vi "niusrprios Open and Configure Device.vi"(0 "USRP RIO Device":T16, 5 "reference frequency source":string(combo)="Internal", 7 "which bitfile":string(combo)="Time", 9 "Wait for GPS Lock?":bool, 11 "error in":errorcluster, 12 "rx config":T4={"rf enable 0"=FALSE, "rf config 0"={"antenna"="RX2", "frequency"=2000000000.0, "lo frequency"=-1.0, "level"=0.0}, "rf enable 1"=FALSE, "rf config 1"={"antenna"="RX2", "frequency"=2000000000.0, "lo frequency"=-1.0, "level"=0.0}, "transfer mode"=enum."Finite", "sample rate"=10000000.0, "number of samples"=8192, "start trigger"=enum."Immediate"} {"sample rate" format="%#.3pS/s"; "rf config 1"."level" format="%#_gdBm"; "rf config 1"."lo frequency" format="%#.3pHz"; "rf config 1"."frequency" format="%#.3pHz"; "rf config 0"."level" format="%#_gdBm"; "rf config 0"."lo frequency" format="%#.3pHz"; "rf config 0"."frequency" format="%#.3pHz"}, 13 "tx config":T5={"rf enable 0"=FALSE, "rf config 0"={"antenna"="TX1", "frequency"=2000000000.0, "lo frequency"=-1.0, "level"=0.0}, "rf enable 1"=FALSE, "rf config 1"={"antenna"="TX1", "frequency"=2000000000.0, "lo frequency"=-1.0, "level"=0.0}, "transfer mode"=enum."Finite", "sample rate"=10000000.0, "number of samples"=8192, "start trigger"=enum."Immediate", "tone frequency"=100000.0} {"tone frequency" format="%#.3pHz"; "sample rate" format="%#.3pS/s"; "rf config 0"."level" format="%#_gdBm"; "rf config 0"."lo frequency" format="%#.3pHz"; "rf config 0"."frequency" format="%#.3pHz"; "rf config 1"."level" format="%#_gdBm"; "rf config 1"."lo frequency" format="%#.3pHz"; "rf config 1"."frequency" format="%#.3pHz"}) -> (2 "rx channels":T3={"rx config"={"rf enable 0"=FALSE, "rf config 0"={"antenna"="RX2", "frequency"=2000000000.0, "lo frequency"=-1.0, "level"=0.0}, "rf enable 1"=FALSE, "rf config 1"={"antenna"="RX2", "frequency"=2000000000.0, "lo frequency"=-1.0, "level"=0.0}, "transfer mode"=enum."Finite", "sample rate"=10000000.0, "number of samples"=8192, "start trigger"=enum."Immediate"}, "reference frequency source"="Internal", "rx.enabled channels"=[], "vertical range"=[], "rx.coerced configurations"={"coerced frequencies"=[], "coerced lo frequencies"=[], "coerced levels"=[], "coerced sample rates"=[]}} {"rx.coerced configurations"."coerced sample rates" format="%#.3pS/s"; "rx.coerced configurations"."coerced levels" format="%#.3gdBm"; "rx.coerced configurations"."coerced lo frequencies" format="%#.3pHz"; "rx.coerced configurations"."coerced frequencies" format="%#.3pHz"; "rx config"."sample rate" format="%#.3pS/s"; "rx config"."rf config 1"."level" format="%#_gdBm"; "rx config"."rf config 1"."lo frequency" format="%#.3pHz"; "rx config"."rf config 1"."frequency" format="%#.3pHz"; "rx config"."rf config 0"."level" format="%#_gdBm"; "rx config"."rf config 0"."lo frequency" format="%#.3pHz"; "rx config"."rf config 0"."frequency" format="%#.3pHz"; "vertical range" format="%#.3pVpp"}, 3 "tx channels":T2={"tx config"={"rf enable 0"=FALSE, "rf config 0"={"antenna"="TX1", "frequency"=2000000000.0, "lo frequency"=-1.0, "level"=0.0}, "rf enable 1"=FALSE, "rf config 1"={"antenna"="TX1", "frequency"=2000000000.0, "lo frequency"=-1.0, "level"=0.0}, "transfer mode"=enum."Finite", "sample rate"=10000000.0, "number of samples"=8192, "start trigger"=enum."Immediate", "tone frequency"=100000.0}, "reference frequency source"="Internal", "tx.enabled channels"=[], "I"=[], "Q"=[], "tx.coerced configurations"={"coerced frequencies"=[], "coerced lo frequencies"=[], "coerced levels"=[], "coerced sample rates"=[]}} {"tx.coerced configurations"."coerced sample rates" format="%#.3pS/s"; "tx.coerced configurations"."coerced levels" format="%#.3gdBm"; "tx.coerced configurations"."coerced lo frequencies" format="%#.3pHz"; "tx.coerced configurations"."coerced frequencies" format="%#.3pHz"; "tx config"."tone frequency" format="%#.3pHz"; "tx config"."sample rate" format="%#.3pS/s"; "tx config"."rf config 0"."level" format="%#_gdBm"; "tx config"."rf config 0"."lo frequency" format="%#.3pHz"; "tx config"."rf config 0"."frequency" format="%#.3pHz"; "tx config"."rf config 1"."level" format="%#_gdBm"; "tx config"."rf config 1"."lo frequency" format="%#.3pHz"; "tx config"."rf config 1"."frequency" format="%#.3pHz"}, 4 "niUsrpRio Session (out)":T7 {"Daughterboard Clock Rate" format="%#.3pHz"; "FPGA Data Clock Rate" format="%#.3pHz"; "Data Clock Rate" format="%#.3pHz"; "Characterization Data"."Frequencies [Hz]" format="%#_6p"; "EEPROM Characterization Header"."Pointer to Device Data Header" format="%x"; "EEPROM Characterization Header"."Checksum" format="%x"; "Device Data Header"."Pointer to Characterization Data" format="%x"; "Device Data Header"."Checksum" format="%x"; "EEPROM Header"."Pointer to User Header" format="%x"; "EEPROM Header"."Pointer to Factory Header" format="%x"; "EEPROM Header"."Product Code" format="%x"; "EEPROM Header"."Checksum" format="%x"}, 6 "rx.coerced configurations":T6 {"coerced sample rates" format="%#.3pS/s"; "coerced levels" format="%#.3gdBm"; "coerced lo frequencies" format="%#.3pHz"; "coerced frequencies" format="%#.3pHz"}, 8 "tx.coerced configurations":T6 {"coerced sample rates" format="%#.3pS/s"; "coerced levels" format="%#.3gdBm"; "coerced lo frequencies" format="%#.3pHz"; "coerced frequencies" format="%#.3pHz"}, 10 "tx.output waveform":waveform(dbl)[](graph), 15 "error out":errorcluster)   [LabVIEW 2015]
doc: "Opens a session to the USRP RIO design library, initializes the device and configures the RF components.\n\n<B>Input Parameters</B>\n\n<B>USRP RIO device</B> is the specific device to open a session to.\n\n<B>reference frequency source</B> is the reference source to use for the clocks of the device. The reference frequency must be 10 MHz.\n\n<B>error in</B> describes error conditions that occur before this node runs. This input provides standard 'error in' functionality.\n\n<B>rx config</B> is the set of configuration values for the Rx signal chain.\n\n<B>tx config</B> is the set of configuration values for the Tx signal chain.\n\n<B>Output Parameters</B>\n\n<B>niUsrpRio Session (out)</B> is the niUsrpRio session used in all subsequent USRP RIO design library host VIs.\n\n<B>rx.coerced configurations</B> are the actual configuration values for the Rx signal chain.\n\n<B>tx.coerced configurations</B> are the actual configuration values for the Tx signal chain.\n\n<B>tx.output waveform</B> is the baseband signal to use when transmitting.\n\n<B>error out</B> contains error information. This output provides standard 'error out' functionality."
uses:
  <vilib>/userdefined/Silver/nirio_resource_slv.ctl
  <instrlib>/niUsrpRio/Config/v1/Host/Public/niUsrpRio Session.ctl
  <instrlib>/_niInstr/Register Bus/v0/Host/Public/Register Bus Session.ctl
  <instrlib>/_niInstr/Register Bus/v0/Host/Private/Session Data.ctl
  <instrlib>/niUsrpRio/Config/v1/Host/Private/DB Queue Reference.ctl
  <instrlib>/niUsrpRio/Config/v1/Host/Private/Daughterboard Data.ctl
  <instrlib>/niUsrpRio/Config/v1/Host/Private/ATR state data.ctl
  <instrlib>/niUsrpRio/Config/v1/Host/Private/Antenna Configuration.ctl
  <instrlib>/niUsrpRio/Config/v1/Host/Private/CPLD Power Mode.ctl
  <instrlib>/niUsrpRio/Config/v1/Host/Public/EEPROM Header.ctl
  <instrlib>/niUsrpRio/Config/v1/Host/Public/EEPROM Device Data Header.ctl
  <instrlib>/niUsrpRio/Config/v1/Host/Public/EEPROM Characterization Header.ctl
  <instrlib>/niUsrpRio/Config/v1/Host/Public/Characterization Data.ctl
  <instrlib>/niUsrpRio/Config/v1/Host/Public/IQ Imbalance.ctl
  niusrprios Start Trigger.ctl
  <instrlib>/_niInstr/Register Bus/v0/Host/niInstr Register Bus v0 Host.lvlib
  <instrlib>/niUsrpRio/Config/v1/Host/niUsrpRio Config v1 Host.lvlib
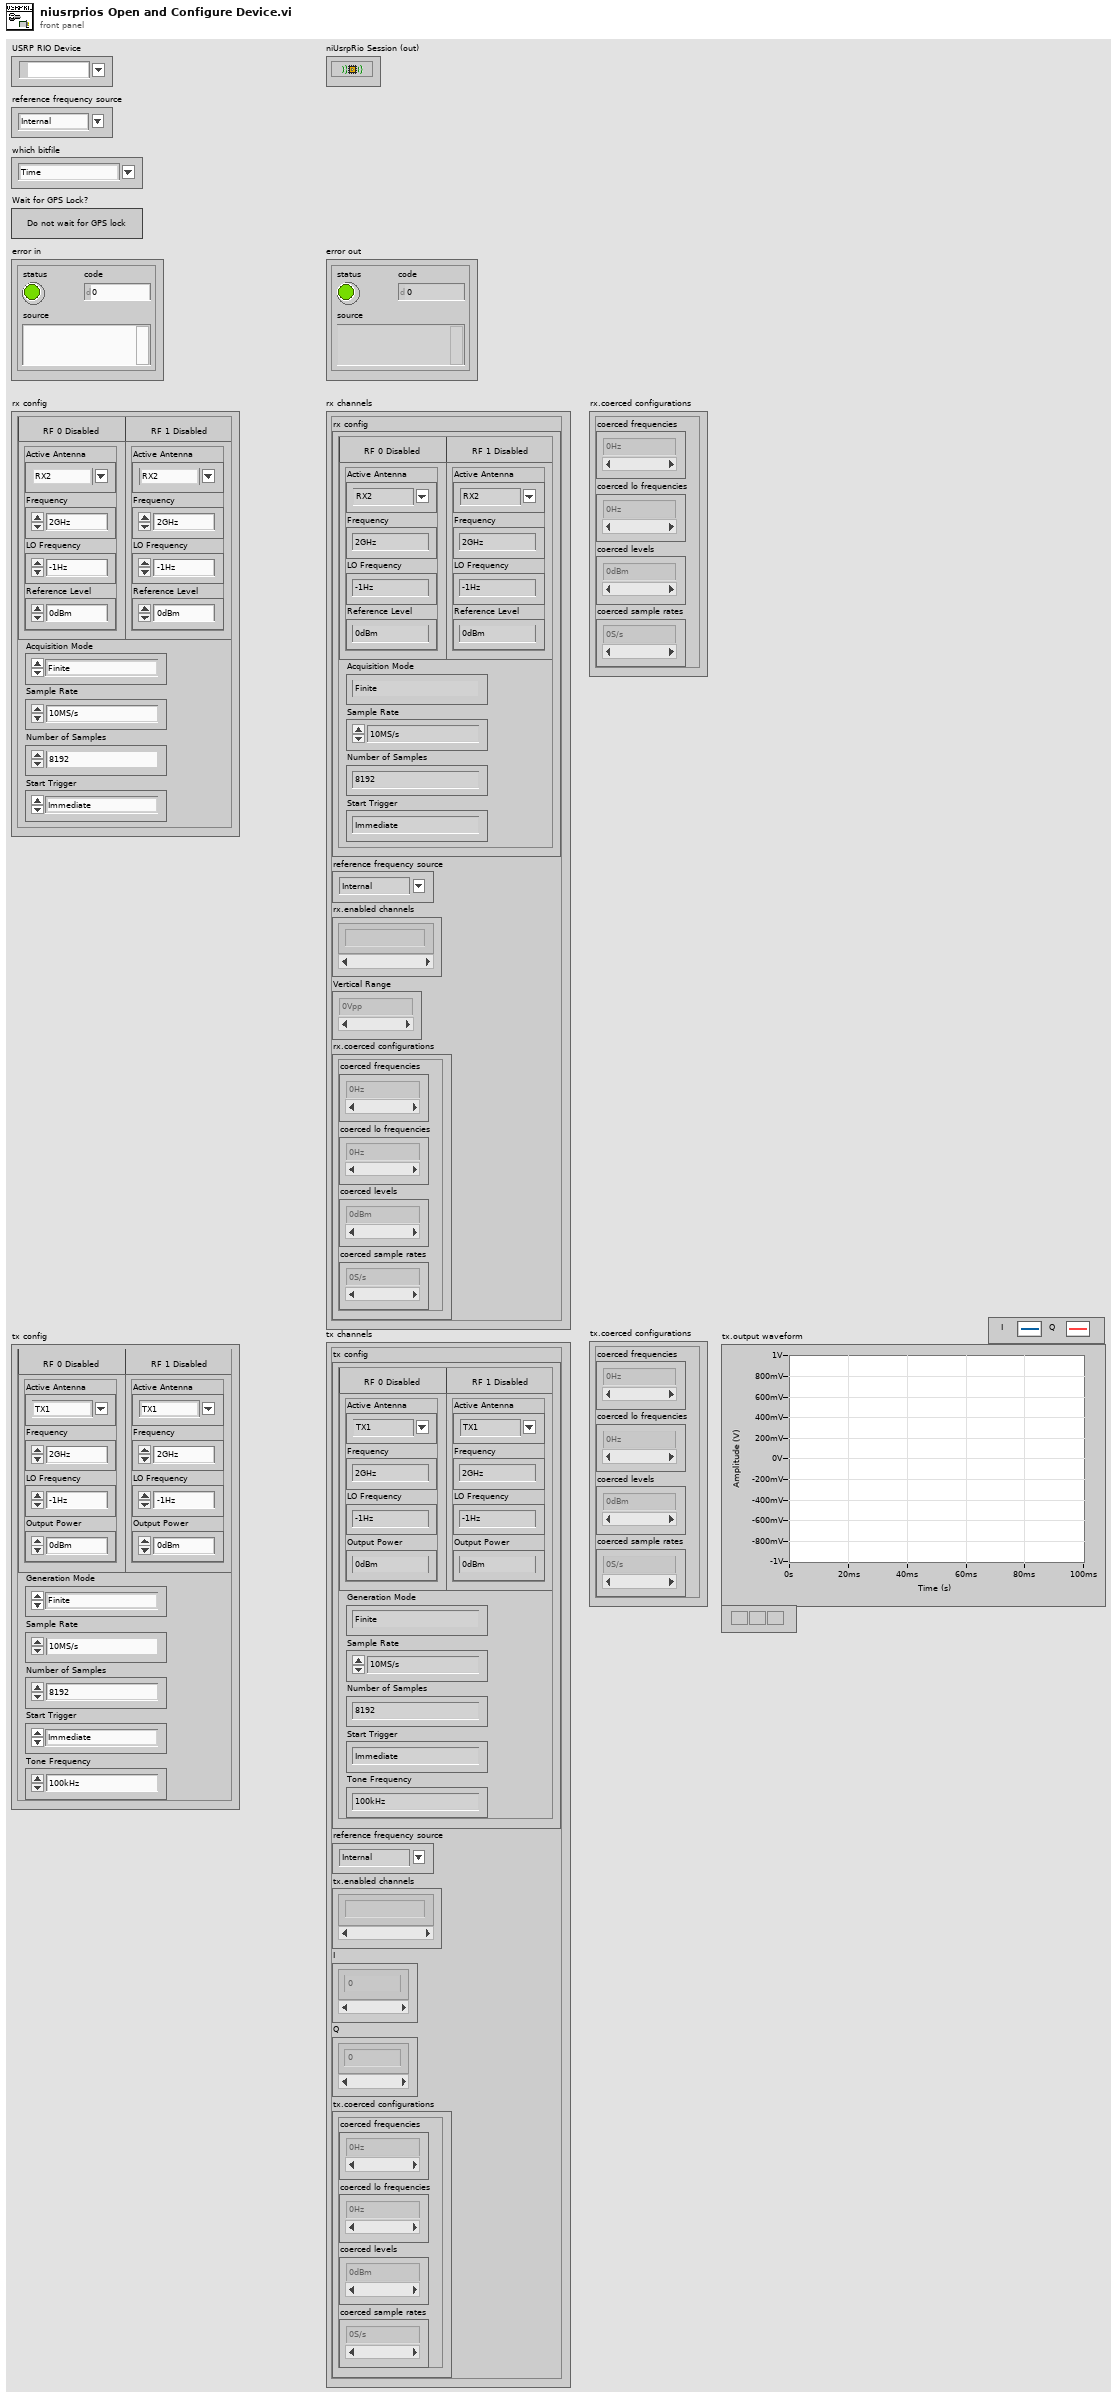
[diagram p1: front panel]
types:
  T1 = typedef "niusrprios Start Trigger.ctl" = enum8{"Software", "Digital Edge", "Rx Start Trigger", "Tx Start Trigger", "Immediate", "Future Time Event"}
  T2 = cluster{"tx config":cluster{"rf enable 0":bool, "rf config 0":cluster{"antenna":string, "frequency":dbl, "lo frequency":dbl, "level":dbl}, "rf enable 1":bool, "rf config 1":cluster{"antenna":string, "frequency":dbl, "lo frequency":dbl, "level":dbl}, "transfer mode":enum16{"Finite", "Continuous"}, "sample rate":dbl, "number of samples":u32, "start trigger":T1, "tone frequency":dbl}, "reference frequency source":string, "tx.enabled channels":string[], "I":i16[], "Q":i16[], "tx.coerced configurations":cluster{"coerced frequencies":dbl[], "coerced lo frequencies":dbl[], "coerced levels":dbl[], "coerced sample rates":dbl[]}}
  T3 = cluster{"rx config":cluster{"rf enable 0":bool, "rf config 0":cluster{"antenna":string, "frequency":dbl, "lo frequency":dbl, "level":dbl}, "rf enable 1":bool, "rf config 1":cluster{"antenna":string, "frequency":dbl, "lo frequency":dbl, "level":dbl}, "transfer mode":enum16{"Finite", "Continuous"}, "sample rate":dbl, "number of samples":u32, "start trigger":T1}, "reference frequency source":string, "rx.enabled channels":string[], "vertical range":dbl[], "rx.coerced configurations":cluster{"coerced frequencies":dbl[], "coerced lo frequencies":dbl[], "coerced levels":dbl[], "coerced sample rates":dbl[]}}
  T4 = cluster{"rf enable 0":bool, "rf config 0":cluster{"antenna":string, "frequency":dbl, "lo frequency":dbl, "level":dbl}, "rf enable 1":bool, "rf config 1":cluster{"antenna":string, "frequency":dbl, "lo frequency":dbl, "level":dbl}, "transfer mode":enum16{"Finite", "Continuous"}, "sample rate":dbl, "number of samples":u32, "start trigger":T1}
  T5 = cluster{"rf enable 0":bool, "rf config 0":cluster{"antenna":string, "frequency":dbl, "lo frequency":dbl, "level":dbl}, "rf enable 1":bool, "rf config 1":cluster{"antenna":string, "frequency":dbl, "lo frequency":dbl, "level":dbl}, "transfer mode":enum16{"Finite", "Continuous"}, "sample rate":dbl, "number of samples":u32, "start trigger":T1, "tone frequency":dbl}
  T6 = cluster{"coerced frequencies":dbl[], "coerced lo frequencies":dbl[], "coerced levels":dbl[], "coerced sample rates":dbl[]}
  T7 = typedef "niUsrpRio Config v1 Host.lvlib/niUsrpRio Session.ctl" = cluster{"FPGA Interface":refnum<k20>, "RIO Interface Number":u32, "Data Clock Rate":u32, "FPGA Data Clock Rate":u32, "Global Settings Register Bus":T8, "Radio 0 Settings Register Bus":T8, "Radio 1 Settings Register Bus":T8, "Radio Settings Bus Semaphore":T9, "DB Queues":T10[], "Characterization Data Valid?":bool, "EEPROM Header":T11, "Device Data Header":T12, "EEPROM Characterization Header":T13, "Characterization Data":T14[], "FPGA Current Version":u32, "FPGA Oldest Compatible Version":u32, "Fixed Logic Current Version":u32, "Fixed Logic Oldest Compatible Version":u32, "FPGA Radio Settings Bus Current Version":u32, "FPGA Radio Settings Bus Oldest Compatible Version":u32, "FPGA Board Config Current Version":u32, "FPGA Board Config Oldest Compatible Version":u32, "Daughterboard Clock Rate":u32}
  T8 = typedef "niInstr Register Bus v0 Host.lvlib/Register Bus Session.ctl" = refnum<queue>
  T9 = typedef "Semaphore RefNum" = refnum<k1>
  T10 = typedef "niUsrpRio Config v1 Host.lvlib/DB Queue Reference.ctl" = refnum<queue>
  T11 = typedef "niUsrpRio Config v1 Host.lvlib/EEPROM Header.ctl" = cluster{"Checksum":u32, "Product Code":u16, "Hardware Current Version":u16, "Hardware Oldest Compatible Version":u16, "EEPROM Map Current Version":u16, "EEPROM Map Oldest Compatible Version":u16, "User Password":string, "Pointer to Factory Header":u32, "Pointer to User Header":u32, "Recommended Interval":u16, "Number of Reserved Bytes":i32, "Number of Daughterboards":u8, "Daughterboard IDs":u16[], "Daughterboard Serial Numbers":string[]}
  T12 = typedef "niUsrpRio Config v1 Host.lvlib/EEPROM Device Data Header.ctl" = cluster{"Checksum":u32, "Number of Channels":u8, "Number of Gain Settings":u16[], "Pointer to Characterization Data":u32[], "Number of Reserved Bytes":i32, "Number of Frequencies":u16[]}
  T13 = typedef "niUsrpRio Config v1 Host.lvlib/EEPROM Characterization Header.ctl" = cluster{"Checksum":u32, "Date":timestamp, "Temperature":sgl, "Misc. Info":string, "Pointer to Device Data Header":u32, "Number of Reserved Bytes":i32}
  T14 = typedef "niUsrpRio Config v1 Host.lvlib/Characterization Data.ctl" = cluster{"Gains[dB]":dbl[], "Frequencies [Hz]":dbl[], "IQ Imbalance Table":T15[], "Measured Gains[dB]":dbl[][]}
  T15 = typedef "niUsrpRio Config v1 Host.lvlib/IQ Imbalance.ctl" = cluster{"Gain Imbalance [linear]":dbl, "Phase Imbalance [radians]":dbl, "Offset":cdb}
  T16 = typedef "nirio_resource_slv.ctl" = tag
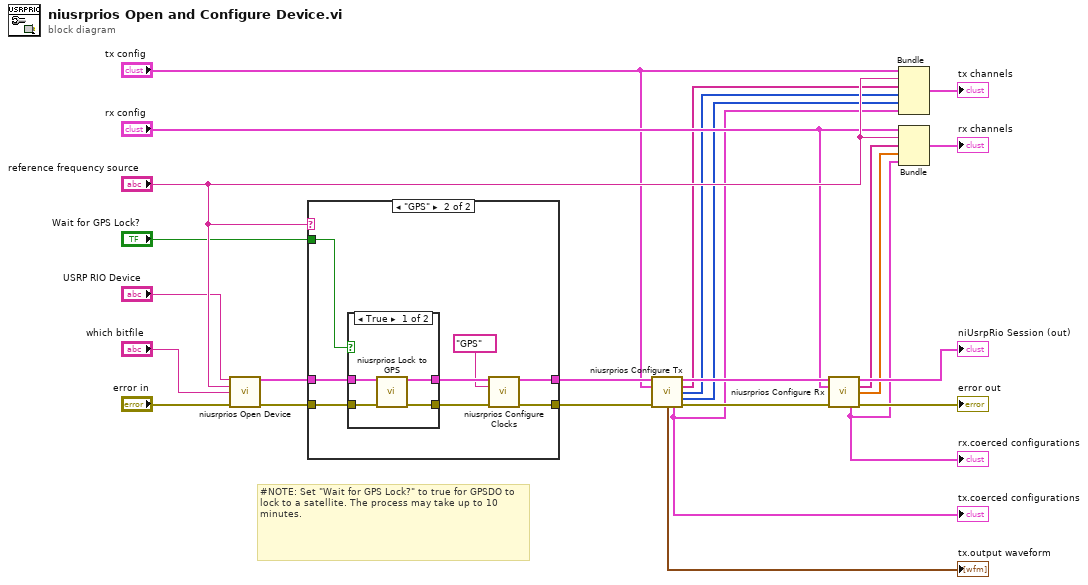
[diagram p0: block diagram]
diagram:
  # "#NOTE: Set \"Wait for GPS Lock?\" to true for GPSDO to lock to a satellite. The process may take up to 10 minutes."
  n1 = call "niusrprios Open Device.vi"("USRP RIO device"="USRP RIO Device", "Reference Frequency Source"="reference frequency source", "which bitfile"="which bitfile", "error in"="error in") -> ("niUsrpRio Session (out)"=w15:T7, "error out"=w16:errorcluster)  [unwired: 10 in]
  n2 = case shown="\"GPS\"" "reference frequency source" {
    tunnel: w15 -> [w27 w35]
    tunnel: [w27 w30] -> w22
    tunnel: [w26 w32] -> w13
    tunnel: w16 -> [w26 w34]
    tunnel: "Wait for GPS Lock?" -> [_ w28]
    frame Default {
    }
    frame "GPS" {
      n3 = case shown="True" w28 {
        tunnel: w35 -> [w37 w41]
        tunnel: [w39 w41] -> w31
        tunnel: [w38 w40] -> w33
        tunnel: w34 -> [w36 w40]
        frame True {
          n4 = call "niusrprios Lock to GPS.vi"("niUsrpRio Session"=w37, "error in"=w36) -> ("niUsrpRio Session (out)"=w39:T7, "error out"=w38:errorcluster)  [unwired: 12 in]
        }
        frame False {
        }
      }
      n5 = call "niusrprios Configure Clocks.vi"("niUsrpRio Session"=w31, "Reference Frequency Source"="GPS", "error in"=w33) -> ("niUsrpRio Session (out)"=w30:T7, "error out"=w32:errorcluster)  [unwired: 11 in]
    }
  }
  n6 = call "niusrprios Configure Tx.vi"("niUsrpRio Session"=w22, "tx config"="tx config", "error in"=w13) -> ("niUsrpRio Session (out)"=w25:T7, "tx.enabled channels"=w9:string[], "I"=w8:i16[], "Q"=w7:i16[], "tx.output waveform"=→"tx.output waveform":waveform(dbl)[], "tx.coerced configurations"=w2:T6, "error out"=w3:errorcluster)  [unwired: 6 in]
  "tx.coerced configurations" <- w2
  n7 = call "niusrprios Configure Rx.vi"("niUsrpRio Session"=w25, "rx config"="rx config", "error in"=w3) -> ("niUsrpRio Session (out)"=→"niUsrpRio Session (out)":T7, "rx.enabled channels"=w11:string[], "vertical range"=w10:dbl[], "rx.coerced configurations"=w1:T6, "error out"=→"error out":errorcluster)  [unwired: 8 in]
  "rx.coerced configurations" <- w1
  n8 = Bundle("tx config"="tx config", "reference frequency source"="reference frequency source", "tx.enabled channels"=w9, "I"=w8, "Q"=w7, "tx.coerced configurations"=w2) -> (→"tx channels":T2)  [unwired: 1 in]
  n9 = Bundle("rx config"="rx config", "reference frequency source"="reference frequency source", "rx.enabled channels"=w11, "vertical range"=w10, "rx.coerced configurations"=w1) -> (→"rx channels":T3)  [unwired: 1 in]
